vi "BME_DG_ReadStatus.vi"(8 "error in (no error)":errorcluster, 11 "DG_Number":i32) -> (0 "error out":errorcluster, 3 "return value":i32)   [LabVIEW 2009]
uses:
  BME Beispiele/BME DLL/DelayGenerator.dll
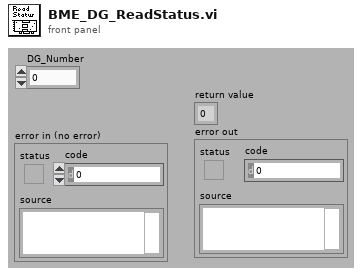
[diagram p1: front panel]
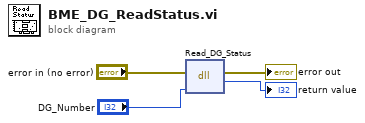
[diagram p0: block diagram]
diagram:
  n1 = dll-call lib="C:/Dokumente und Einstellungen/A2.5/Desktop/BME Beispiele/BME DLL/DelayGenerator.dll" fn="Read_DG_Status"(error in="error in (no error)", "DG_Number"="DG_Number") -> (error out=→"error out":errorcluster, "return type"=→"return value":i32)  [unwired: 3 in, 1 out]
